vi "Pump_API_ContiFlow_Test.vi"() -> ()   [LabVIEW 2021]
uses:
  labbCAN_Pump_API/VolumeUnits.ctl
  labbCAN_Bus_API/SiUnitPrefix.ctl
  labbCAN_Bus_API/TimeUnits.ctl
  labbCAN_Pump_API/ContiFlowProperties.ctl
  labbCAN_Pump_API/ContiFlowSwitchingModes.ctl
  labbCAN_Bus_API/labbCAN_Bus_API.lvlib
  labbCAN_Pump_API/labbCAN_Pump_API.lvlib
  labbCAN_Valve_API/labbCAN_Valve_API.lvlib
panel:
  out "Status":string="Test 5: Continuous flow dosage"
  out "Maximum Flow Rate":dbl
  out "Test Step:":string
  out "error out":errorcluster
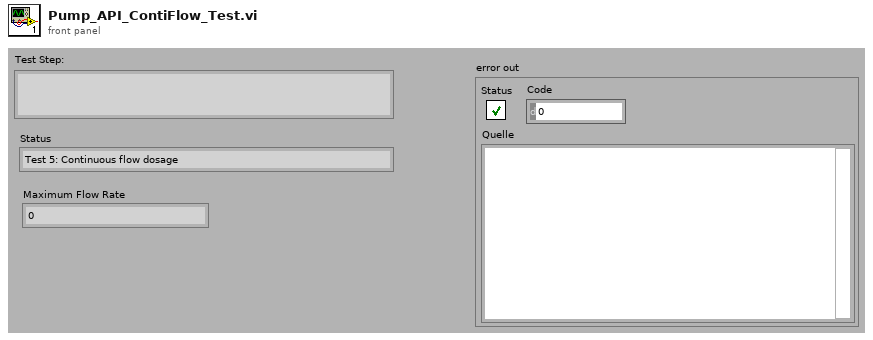
[diagram p1: front panel]
types:
  T1 = cluster{"hValve":i64, "AspiratingPos":i32, "DispensingPos":i32, "ClosedPos":i32}
  T2 = typedef "labbCAN_Bus_API.lvlib/TimeUnits.ctl" = i32
  T3 = typedef "labbCAN_Pump_API.lvlib/VolumeUnits.ctl" = i32
  T4 = typedef "labbCAN_Bus_API.lvlib/SiUnitPrefix.ctl" = i32
  T5 = typedef "labbCAN_Pump_API.lvlib/ContiFlowProperties.ctl" = u8
  T6 = typedef "labbCAN_Pump_API.lvlib/ContiFlowSwitchingModes.ctl" = u8
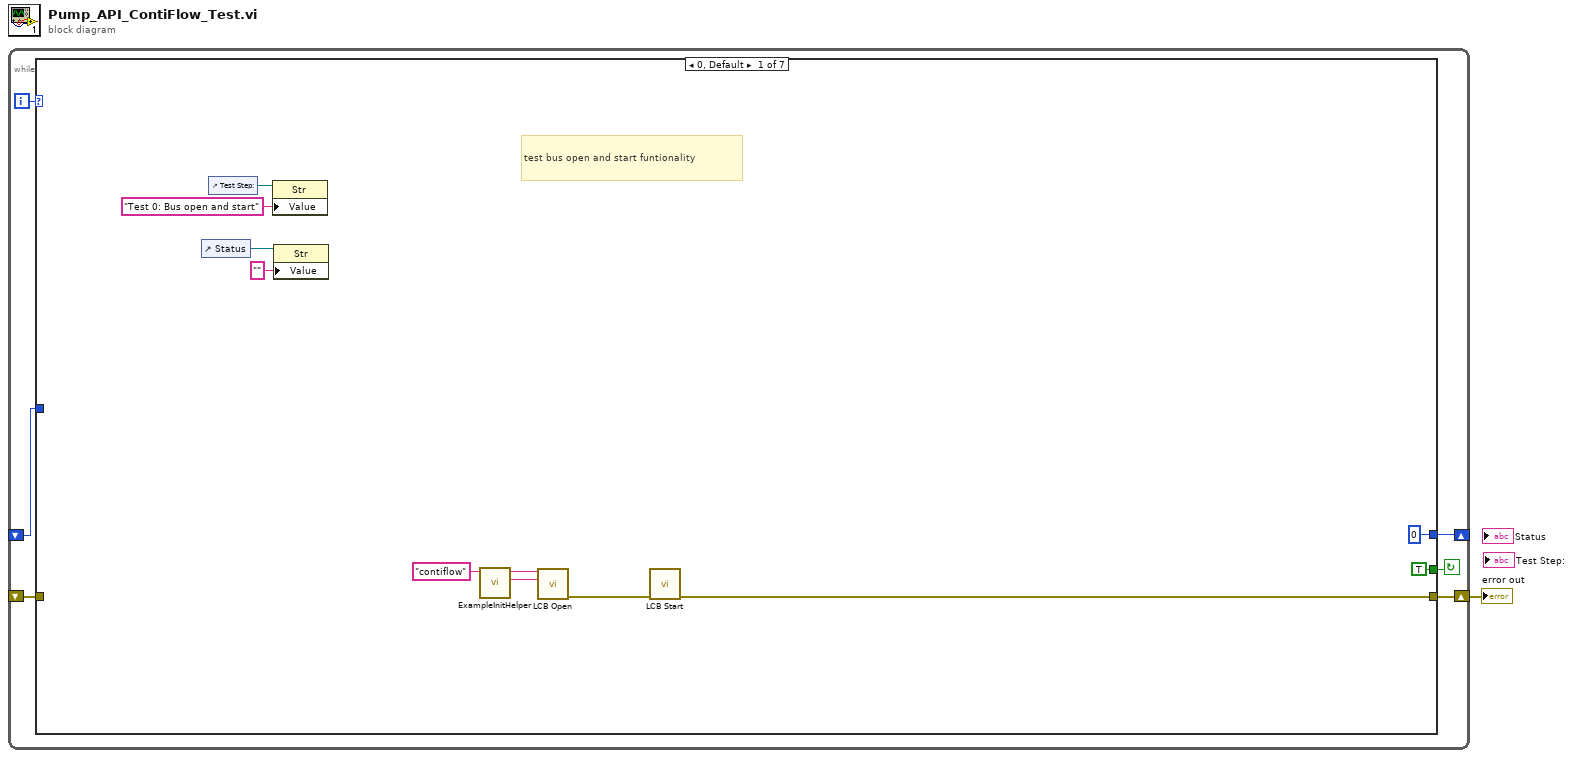
[diagram p0: block diagram]
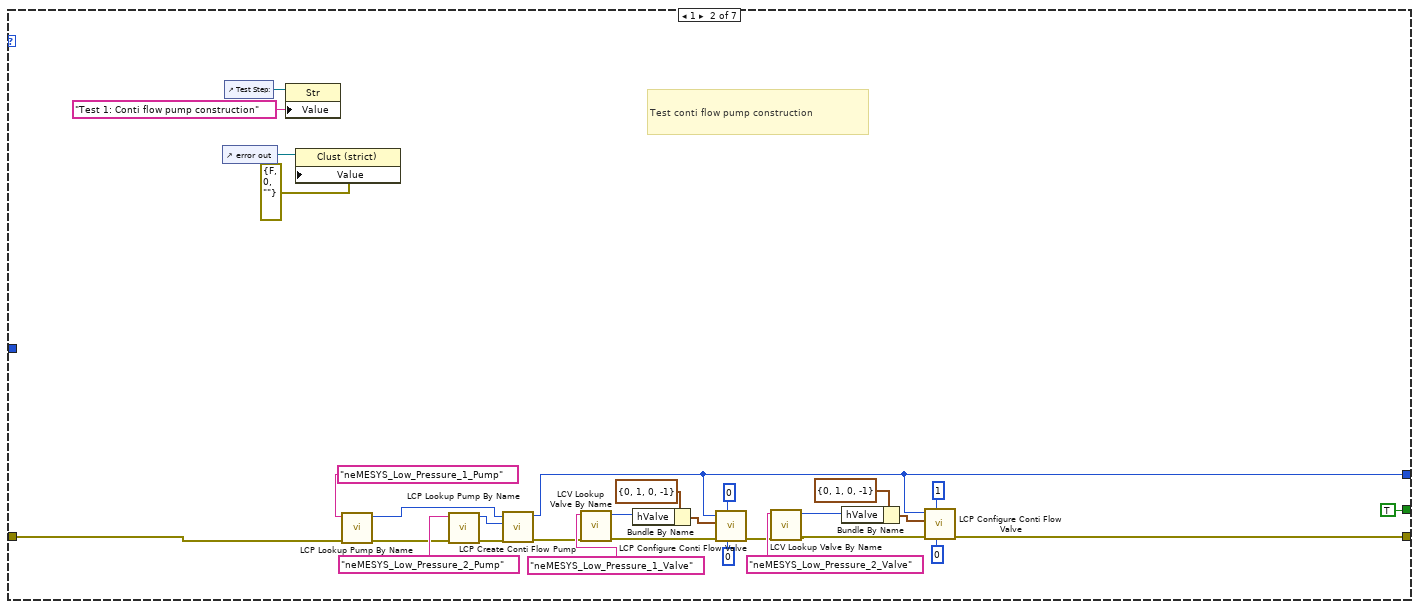
[diagram p2: hidden frame]
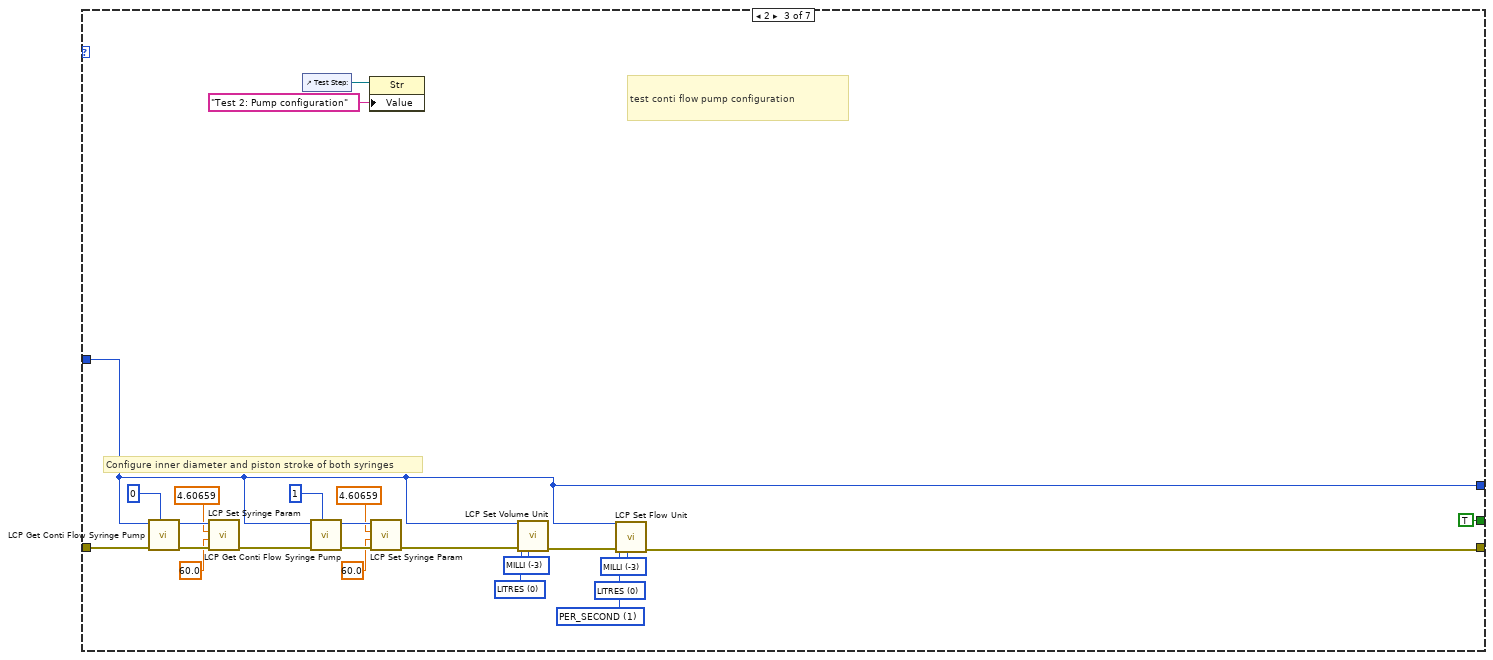
[diagram p3: hidden frame]
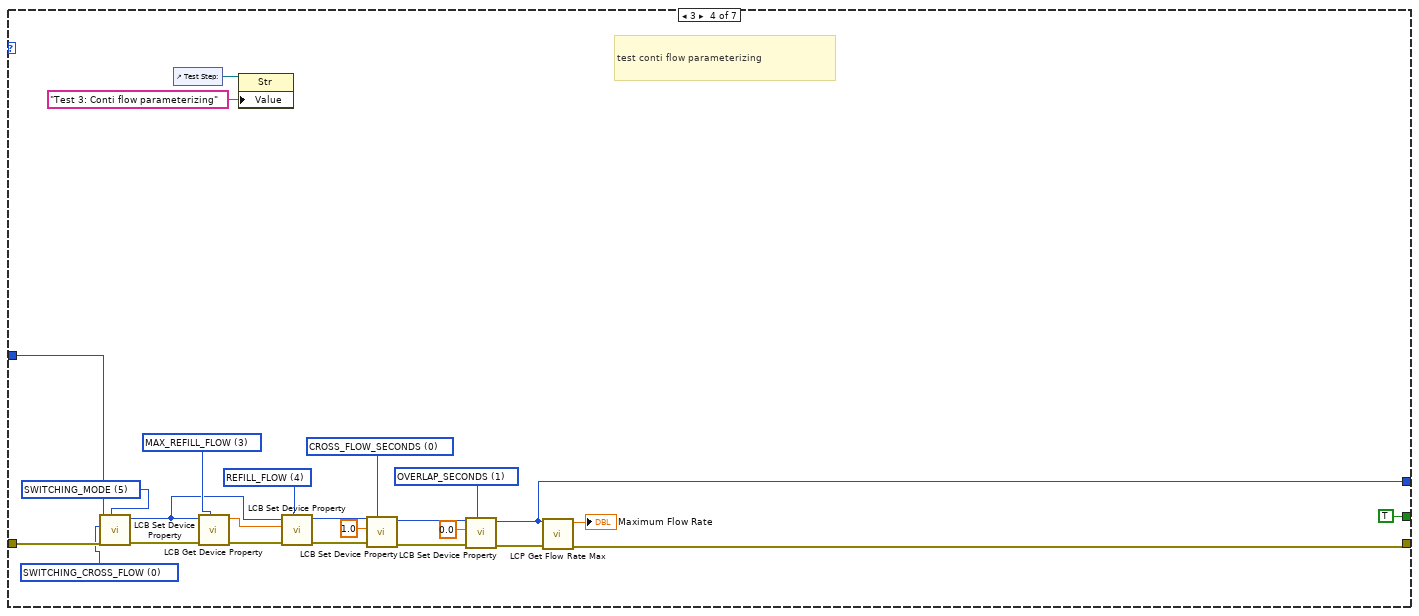
[diagram p4: hidden frame]
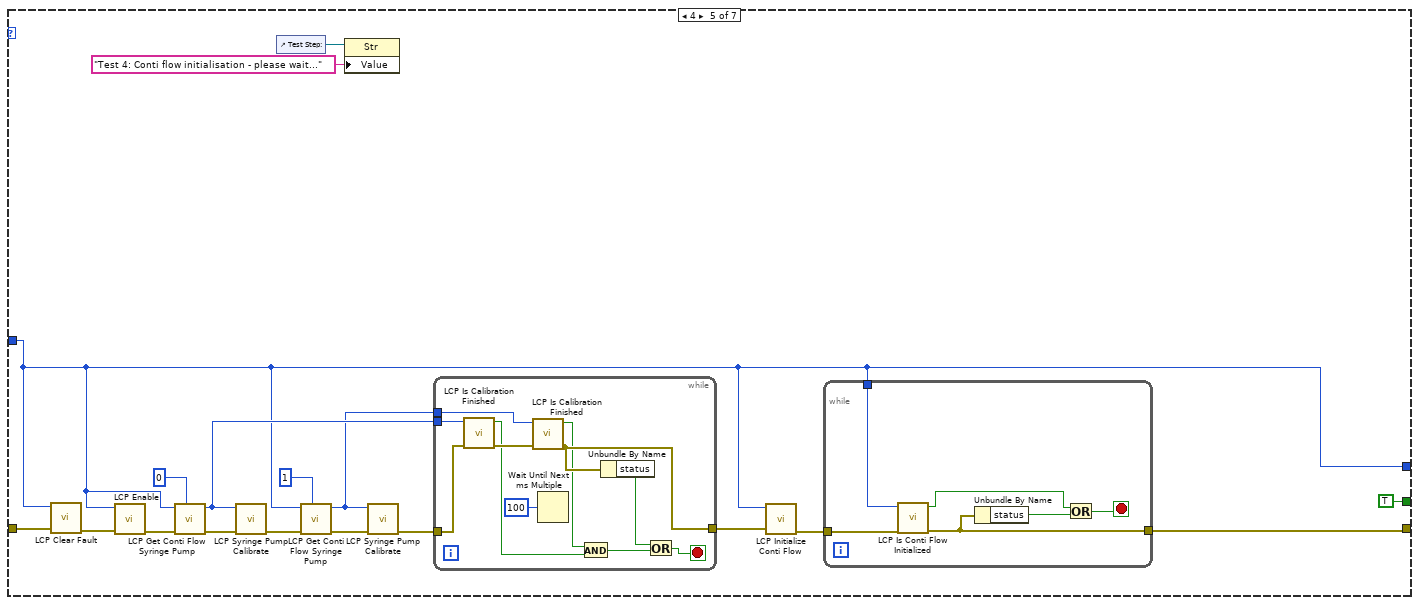
[diagram p5: hidden frame]
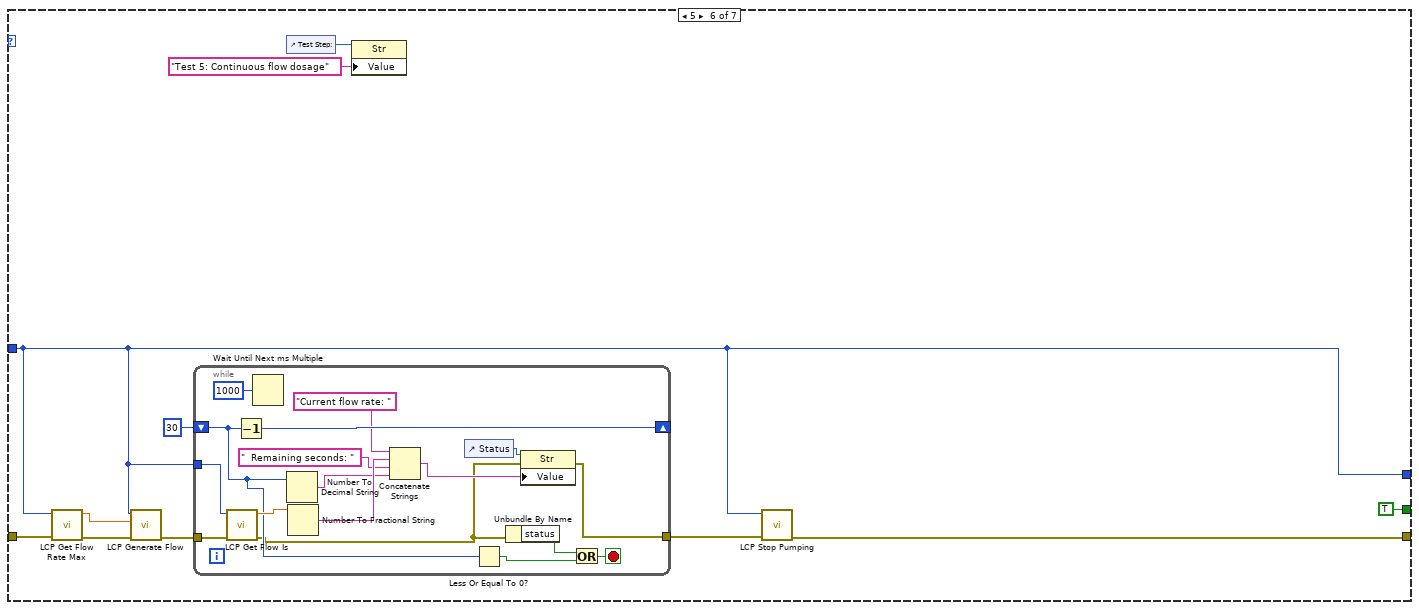
[diagram p6: hidden frame]
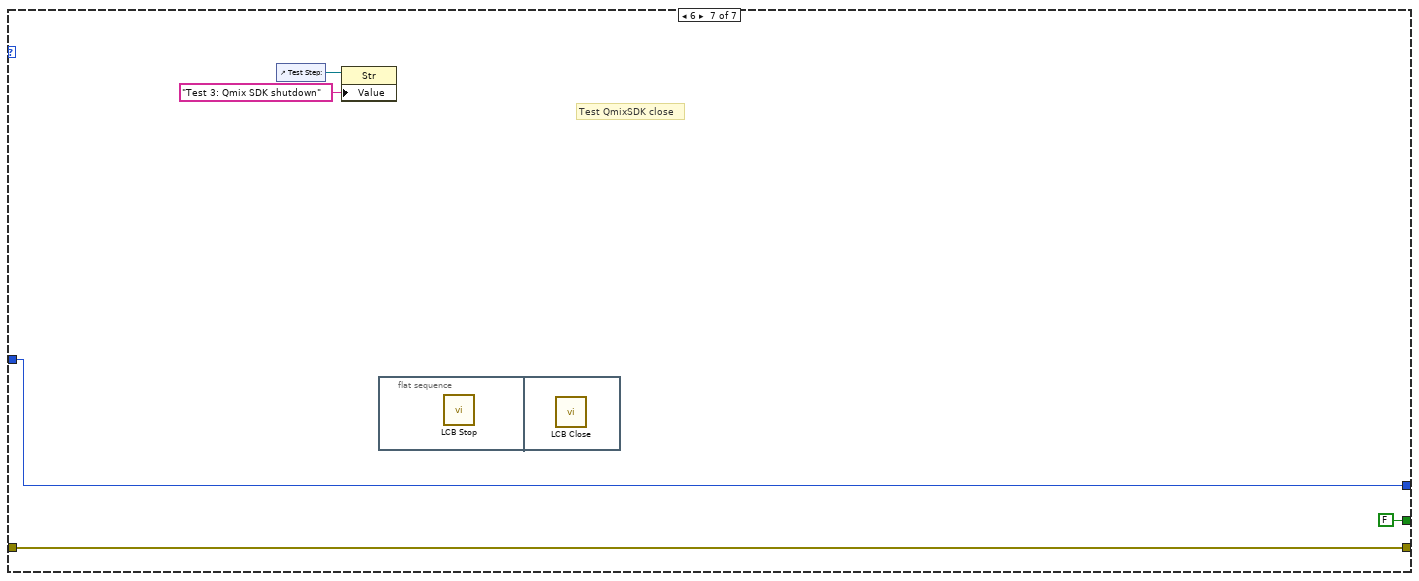
[diagram p7: hidden frame]
diagram:
  n1 = while {
    shift-right: [w4] -> w1
    shift-left: _ -> [w5]
    shift-right: [w3] -> _
    shift-left: _ -> [w2]
    i -> [w7]
    stop <- w6 continue-if-true
    n2 = case shown="0, Default" w7 {
      tunnel: [TRUE TRUE TRUE TRUE TRUE TRUE FALSE] -> w6
      tunnel: w5 -> [_ w27 w71 w97 w115 w141 w161]
      tunnel: [w16 w26 w52 w78 w98 w135 w161] -> w4
      tunnel: [i64 0 ("ContiFlowPumpHandle") w25 w51 w77 w99 w134 w164] -> w3
      tunnel: w2 -> [_ _ w51 w90 w99 w134 w164]
      frame 0, Default {
        # "test bus open and start funtionality"
        n3 = control-ref of="Status"() -> (w12:refnum<vi>)
        n4 = control-ref of="Test Step:"() -> (w14:refnum<vi>)
        n5 = property class="Str"(reference=w14, "Value"="Test 0: Bus open and start" ("Wert")) -> ()  [unwired: 1 in, 2 out]
        n6 = property class="Str"(reference=w12, "Value"="" ("Wert")) -> ()  [unwired: 1 in, 2 out]
        n7 = call "ExampleInitHelper.vi"("Device Config Name"="contiflow") -> ("Plugin Search Path"=w9:string, "Device Configuration Path"=w10:string)  [unwired: 5 in]
        n8 = call "LCB Open.vi"("PluginSearchPath"=w9, "Device Configuration Path"=w10) -> ("error out"=w17:errorcluster)  [unwired: 9 in]
        n9 = call "LCB Start.vi"("error in (no error)"=w17) -> ("error out"=w16:errorcluster)  [unwired: 10 in]
      }
      frame 1 {
        # "Test conti flow pump construction"
        n10 = control-ref of="error out"() -> (w20:refnum<vi>)
        n11 = control-ref of="Test Step:"() -> (w24:refnum<vi>)
        n12 = property class="Str"(reference=w24, "Value"="Test 1: Conti flow pump construction" ("Wert")) -> ()  [unwired: 1 in, 2 out]
        n13 = property class="Clust (strict)"(reference=w20, "Value"=errorcluster {"status"=FALSE, "code"=0, "source"=""} ("Wert")) -> ()  [unwired: 1 in, 2 out]
        n14 = call "LCP Lookup Pump By Name.vi"("error in (no error)"=w27, "Pump Name"="neMESYS_Low_Pressure_1_Pump" ("pAxisName")) -> ("error out"=w38:errorcluster, "Pump handle"=w22:i64)  [unwired: 8 in]
        n15 = call "LCP Lookup Pump By Name.vi"("error in (no error)"=w38, "Pump Name"="neMESYS_Low_Pressure_2_Pump" ("pAxisName")) -> ("error out"=w37:errorcluster, "Pump handle"=w21:i64)  [unwired: 8 in]
        n16 = call "LCP Create Conti Flow Pump.vi"("error in (no error)"=w37, "SyringePump2"=w21, "SyringePump1"=w22) -> ("error out"=w36:errorcluster, "ContiFlowPumpHandle"=w25:i64)  [unwired: 7 in]
        n17 = call "LCV Lookup Valve By Name.vi"("error in (no error)"=w36, "Valve Name"="neMESYS_Low_Pressure_1_Valve" ("pAxisName")) -> ("error out"=w35:errorcluster, "Valve handle"=w42:i64)  [unwired: 8 in]
        n18 = Bundle By Name(cluster=T1 {"hValve"=0, "AspiratingPos"=1, "DispensingPos"=0, "ClosedPos"=-1} ("ValveConfig"), "hValve"=w42) -> (w41:T1)
        n19 = call "LCP Configure Conti Flow Valve.vi"("ValveIndex"=u32 0, "PumpChannelIndex"=u32 0, "error in (no error)"=w35, "ValveConfig"=w41, "ContiFlowPumpHandle"=w25) -> ("error out"=w34:errorcluster)  [unwired: 5 in, 1 out]
        n20 = call "LCV Lookup Valve By Name.vi"("error in (no error)"=w34, "Valve Name"="neMESYS_Low_Pressure_2_Valve" ("pAxisName")) -> ("error out"=w31:errorcluster, "Valve handle"=w30:i64)  [unwired: 8 in]
        n21 = Bundle By Name(cluster=T1 {"hValve"=0, "AspiratingPos"=1, "DispensingPos"=0, "ClosedPos"=-1} ("ValveConfig"), "hValve"=w30) -> (w28:T1)
        n22 = call "LCP Configure Conti Flow Valve.vi"("ValveIndex"=u32 0, "PumpChannelIndex"=u32 1, "error in (no error)"=w31, "ValveConfig"=w28, "ContiFlowPumpHandle"=w25) -> ("error out"=w26:errorcluster)  [unwired: 5 in, 1 out]
      }
      frame 2 {
        w53 = T2 1 items=["PER_SECOND"=1, "PER_MINUTE"=60, "PER_HOUR"=3600] ("TimeUnit")
        w54 = T3 0 items=["LITRES"] ("VolumeUnit")
        w55 = T4 -3 items=["UNIT"=0, "DECI"=-1, "CENTI"=-2, "MILLI"=-3, "MICRO"=-6] ("Prefix")
        w57 = T3 0 items=["LITRES"] ("Volume Unit")
        w58 = T4 -3 items=["UNIT"=0, "DECI"=-1, "CENTI"=-2, "MILLI"=-3, "MICRO"=-6] ("Prefix")
        # "Configure inner diameter and piston stroke of both syringes"
        # "test conti flow pump configuration"
        n23 = call "LCP Get Conti Flow Syringe Pump.vi"("Pump Channel"=u8 0, "error in (no error)"=w71, "Pump Handle"=w51) -> ("error out"=w69:errorcluster, "SyringePumpHandle"=w68:i64)  [unwired: 7 in]
        n24 = call "LCP Set Syringe Param.vi"("error in (no error)"=w69, "Maximum Piston Stroke (mm)"=60.0, "Inner Diameter (mm)"=4.60659, "Pump Handle"=w68) -> ("error out"=w60:errorcluster)  [unwired: 7 in]
        n25 = control-ref of="Test Step:"() -> (w50:refnum<vi>)
        n26 = call "LCP Get Conti Flow Syringe Pump.vi"("Pump Channel"=u8 1, "error in (no error)"=w60, "Pump Handle"=w51) -> ("error out"=w64:errorcluster, "SyringePumpHandle"=w63:i64)  [unwired: 7 in]
        n27 = property class="Str"(reference=w50, "Value"="Test 2: Pump configuration" ("Wert")) -> ()  [unwired: 1 in, 2 out]
        n28 = call "LCP Set Syringe Param.vi"("error in (no error)"=w64, "Maximum Piston Stroke (mm)"=60.0, "Inner Diameter (mm)"=4.60659, "Pump Handle"=w63) -> ("error out"=w59:errorcluster)  [unwired: 7 in]
        n29 = call "LCP Set Volume Unit.vi"("Prefix"=w58, "error in (no error)"=w59, "Volume Unit"=w57, "Pump Handle"=w51) -> ("error out"=w56:errorcluster)  [unwired: 7 in]
        n30 = call "LCP Set Flow Unit.vi"("Prefix"=w55, "error in (no error)"=w56, "TimeUnit"=w53, "VolumeUnit"=w54, "Pump Handle"=w51) -> ("error out"=w52:errorcluster)  [unwired: 6 in]
      }
      frame 3 {
        w81 = T5 1 items=["CROSS_FLOW_SECONDS", "OVERLAP_SECONDS", "MIN_PUMP_FLOW", "MAX_REFILL_FLOW", "REFILL_FLOW", "SWITCHING_MODE"] ("ContiFlowProperties")
        w85 = T5 0 items=["CROSS_FLOW_SECONDS", "OVERLAP_SECONDS", "MIN_PUMP_FLOW", "MAX_REFILL_FLOW", "REFILL_FLOW", "SWITCHING_MODE"] ("ContiFlowProperties")
        w88 = T5 4 items=["CROSS_FLOW_SECONDS", "OVERLAP_SECONDS", "MIN_PUMP_FLOW", "MAX_REFILL_FLOW", "REFILL_FLOW", "SWITCHING_MODE"] ("ContiFlowProperties")
        w93 = T5 3 items=["CROSS_FLOW_SECONDS", "OVERLAP_SECONDS", "MIN_PUMP_FLOW", "MAX_REFILL_FLOW", "REFILL_FLOW", "SWITCHING_MODE"] ("ContiFlowProperties")
        w95 = T6 0 items=["SWITCHING_CROSS_FLOW"] ("ContiFlowSwitchingModes")
        w96 = T5 5 items=["CROSS_FLOW_SECONDS", "OVERLAP_SECONDS", "MIN_PUMP_FLOW", "MAX_REFILL_FLOW", "REFILL_FLOW", "SWITCHING_MODE"] ("ContiFlowProperties")
        # "test conti flow parameterizing"
        n31 = call "LCB Set Device Property.vi"("Property ID"=w96, "error in (no error)"=w97, "Value"=w95, "Device Handle"=w90) -> ("error out"=w94:errorcluster, "Device Handle Out"=w89:i64)  [unwired: 6 in]
        n32 = control-ref of="Test Step:"() -> (w75:refnum<vi>)
        n33 = call "LCB Get Device Property.vi"("Property ID"=w93, "error in (no error)"=w94, "Device Handle"=w89) -> ("error out"=w92:errorcluster, "Property Value"=w91:dbl)  [unwired: 7 in]
        n34 = property class="Str"(reference=w75, "Value"="Test 3: Conti flow parameterizing" ("Wert")) -> ()  [unwired: 1 in, 2 out]
        n35 = call "LCB Set Device Property.vi"("Property ID"=w88, "error in (no error)"=w92, "Value"=w91, "Device Handle"=w89) -> ("error out"=w86:errorcluster, "Device Handle Out"=w87:i64)  [unwired: 6 in]
        n36 = call "LCB Set Device Property.vi"("Property ID"=w85, "error in (no error)"=w86, "Value"=1.0, "Device Handle"=w87) -> ("error out"=w83:errorcluster, "Device Handle Out"=w82:i64)  [unwired: 6 in]
        n37 = call "LCB Set Device Property.vi"("Property ID"=w81, "error in (no error)"=w83, "Value"=0.0, "Device Handle"=w82) -> ("error out"=w79:errorcluster, "Device Handle Out"=w77:i64)  [unwired: 6 in]
        n38 = call "LCP Get Flow Rate Max.vi"("error in (no error)"=w79, "Pump Handle"=w77) -> ("error out"=w78:errorcluster, "Maximum Flow Rate"=→"Maximum Flow Rate":dbl)  [unwired: 8 in]
      }
      frame 4 {
        n39 = call "LCP Clear Fault.vi"("error in (no error)"=w115, "Pump Handle"=w99) -> ("error out"=w114:errorcluster)  [unwired: 9 in]
        n40 = call "LCP Enable.vi"("error in (no error)"=w114, "Pump Handle"=w99) -> ("error out"=w113:errorcluster)  [unwired: 9 in]
        n41 = call "LCP Get Conti Flow Syringe Pump.vi"("Pump Channel"=u8 0, "error in (no error)"=w113, "Pump Handle"=w99) -> ("error out"=w111:errorcluster, "SyringePumpHandle"=w106:i64)  [unwired: 7 in]
        n42 = call "LCP Syringe Pump Calibrate.vi"("error in (no error)"=w111, "Pump Handle"=w106) -> ("error out"=w110:errorcluster)  [unwired: 9 in]
        n43 = control-ref of="Test Step:"() -> (w103:refnum<vi>)
        n44 = call "LCP Get Conti Flow Syringe Pump.vi"("Pump Channel"=u8 1, "error in (no error)"=w110, "Pump Handle"=w99) -> ("error out"=w108:errorcluster, "SyringePumpHandle"=w105:i64)  [unwired: 7 in]
        n45 = property class="Str"(reference=w103, "Value"="Test 4: Conti flow initialisation - please wait..." ("Wert")) -> ()  [unwired: 1 in, 2 out]
        n46 = call "LCP Syringe Pump Calibrate.vi"("error in (no error)"=w108, "Pump Handle"=w105) -> ("error out"=w107:errorcluster)  [unwired: 9 in]
        n47 = while {
          tunnel: w107 -> [w132]
          tunnel: w106 -> [w131]
          tunnel: w105 -> [w129]
          tunnel: [w128] -> w101
          stop <- w122 stop-if-true
          n48 = call "LCP Is Calibration Finished.vi"("error in (no error)"=w132, "Pump Handle"=w131) -> ("error out"=w130:errorcluster, "Calibration Finished"=w127:bool)  [unwired: 8 in]
          n49 = call "LCP Is Calibration Finished.vi"("error in (no error)"=w130, "Pump Handle"=w129) -> ("error out"=w128:errorcluster, "Calibration Finished"=w126:bool)  [unwired: 8 in]
          n50 = Wait Until Next ms Multiple(millisecond multiple=u32 100 ("Vielfache von ms")) -> ()  [unwired: 1 out]
          n51 = And(x=w126, y=w127) -> (x .and. y?=w124:bool)
          n52 = Unbundle By Name(w128) -> ("status"=w123:bool)
          n53 = Or(x=w123, y=w124) -> (x .or. y?=w122:bool)
        }
        n54 = call "LCP Initialize Conti Flow.vi"("error in (no error)"=w101, "ContiFlowPumpHandle"=w99) -> ("error out"=w100:errorcluster)  [unwired: 9 in]
        n55 = while {
          tunnel: w100 -> [w121]
          tunnel: w99 -> [w120]
          tunnel: [w119] -> w98
          stop <- w116 stop-if-true
          n56 = call "LCP Is Conti Flow Initialized.vi"("error in (no error)"=w121, "ContiFlowPumpHandle"=w120) -> ("error out"=w119:errorcluster, "Initialized"=w117:bool)  [unwired: 8 in]
          n57 = Unbundle By Name(w119) -> ("status"=w118:bool)
          n58 = Or(x=w117, y=w118) -> (x .or. y?=w116:bool)
        }
      }
      frame 5 {
        n59 = call "LCP Get Flow Rate Max.vi"("error in (no error)"=w141, "Pump Handle"=w134) -> ("error out"=w140:errorcluster, "Maximum Flow Rate"=w133:dbl)  [unwired: 8 in]
        n60 = call "LCP Generate Flow.vi"("error in (no error)"=w140, "Flow Rate"=w133, "Pump Handle"=w134) -> ("error out"=w139:errorcluster)  [unwired: 8 in]
        n61 = while {
          tunnel: w139 -> [w160]
          tunnel: w134 -> [w157]
          shift-right: [w156] -> _
          shift-left: 30 -> [w148]
          tunnel: [w149] -> w136
          stop <- w146 stop-if-true
          n62 = call "LCP Get Flow Is.vi"("error in (no error)"=w160, "Pump Handle"=w157) -> ("error out"=w147:errorcluster, "Actual Flow Rate"=w158:dbl)  [unwired: 8 in]
          n63 = Decrement(x=w148) -> (x-1=w156:i32)
          n64 = Wait Until Next ms Multiple(millisecond multiple=u32 1000 ("Vielfache von ms")) -> ()  [unwired: 1 out]
          n65 = Number To Decimal String(number=w148) -> (decimal integer string=w152:string)  [unwired: 1 in]
          n66 = Number To Fractional String(number=w158) -> (F-format string=w154:string)  [unwired: 3 in]
          n67 = Concatenate Strings("Current flow rate: " ("String"), w154, "  Remaining seconds: " ("String"), w152) -> (w150:string)
          n68 = control-ref of="Status"() -> (w151:refnum<vi>)
          n69 = Less Or Equal To 0?(x=w148) -> (x <= 0?=w145:bool)
          n70 = Unbundle By Name(w147) -> ("status"=w144:bool)
          n71 = property class="Str"(reference=w151, error in=w147, "Value"=w150) -> (error out=w149:errorcluster)  [unwired: 1 out]
          n72 = Or(x=w144, y=w145) -> (x .or. y?=w146:bool)
        }
        n73 = control-ref of="Test Step:"() -> (w143:refnum<vi>)
        n74 = property class="Str"(reference=w143, "Value"="Test 5: Continuous flow dosage" ("Wert")) -> ()  [unwired: 1 in, 2 out]
        n75 = call "LCP Stop Pumping.vi"("error in (no error)"=w136, "Pump Handle"=w134) -> ("error out"=w135:errorcluster)  [unwired: 9 in]
      }
      frame 6 {
        # "Test QmixSDK close"
        n76 = control-ref of="Test Step:"() -> (w163:refnum<vi>)
        n77 = property class="Str"(reference=w163, "Value"="Test 3: Qmix SDK shutdown" ("Wert")) -> ()  [unwired: 1 in, 2 out]
        n78 = flat-sequence {
          frame #0 {
            n79 = call "LCB Stop.vi"() -> ()  [unwired: 11 in, 1 out]
          }
          frame #1 {
            n80 = call "LCB Close.vi"() -> ()  [unwired: 11 in, 1 out]
          }
        }
      }
    }
  }
  "error out" <- w1
